vi "Ctor.vi"(6 "Element Changed Callback":refnum<vi>, 7 "Callback Owner":refnum<class>, 8 "error in (no error)":errorcluster, 9 "Array":refnum<vi>, 10 "Scrollbar":refnum<vi>, 11 "Controls":refnum<vi>[](array[refnum])) -> (0 "error out":errorcluster, 3 "ControlArray out":refnum<class "ControlArray.lvclass">)   [LabVIEW 2020, in "Control Array.lvlib" / "ControlArray.lvclass"]
uses:
  ControlArray.lvclass
  ControlArray.lvclass/ControlArray.ctl
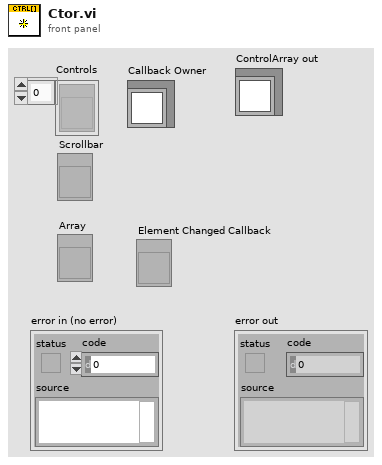
[diagram p1: front panel]
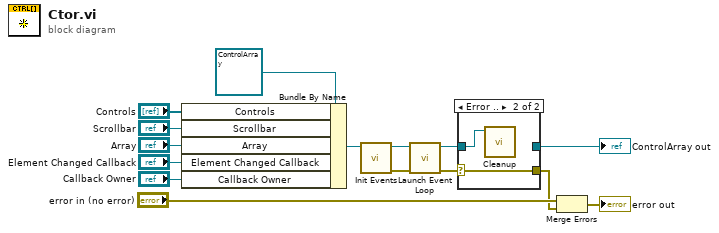
[diagram p0: block diagram]
diagram:
  n1 = Bundle By Name(cluster=refnum<class "ControlArray.lvclass"> refnum ("Control Array.lvlib:ControlArray.lvclass"), "Controls"="Controls", "Scrollbar"="Scrollbar", "Array"="Array", "Element Changed Callback"="Element Changed Callback", "Callback Owner"="Callback Owner") -> (w1:refnum<class "ControlArray.lvclass">)
  n2 = call "Init Events.vi"("ControlArray in"=w1) -> ("error out"=w9:errorcluster, "ControlArray out"=w10:refnum<class "ControlArray.lvclass">)  [unwired: 9 in]
  n3 = call "Launch Event Loop.vi"("error in (no error)"=w9, "ControlArray in"=w10) -> ("error out"=w8:errorcluster, "ControlArray out"=w7:refnum<class "ControlArray.lvclass">)  [unwired: 8 in]
  n4 = case shown="Error .." w8 {
    selector: w8 -> [w16 w18]
    tunnel: w7 -> [w17 w19]
    tunnel: [w17 _] -> w6
    tunnel: [w16 w18] -> w3
    frame No Error {
    }
    frame Error {
      n5 = call "Cleanup.vi"("ControlArray in"=w19) -> ()  [unwired: 10 in, 1 out]
    }
  }
  "ControlArray out" <- w6
  n6 = Merge Errors("error in (no error)", w3) -> (→"error out":errorcluster)
